vi "Prime95BCameraSimpleOperation.vi"(8 "error in (no error)":errorcluster, 11 "Config In":T3 {"Hardware Configuration"."Lasers Configuration"."SettingValues"."785 Power" format="%.1f"; "Hardware Configuration"."Lasers Configuration"."SettingValues"."647 Power" format="%.1f"; "Hardware Configuration"."Lasers Configuration"."SettingValues"."561 Power" format="%.1f"}) -> (0 "error out":errorcluster, 3 "Config Out":T3 {"Hardware Configuration"."Lasers Configuration"."SettingValues"."785 Power" format="%.1f"; "Hardware Configuration"."Lasers Configuration"."SettingValues"."647 Power" format="%.1f"; "Hardware Configuration"."Lasers Configuration"."SettingValues"."561 Power" format="%.1f"})   [LabVIEW 2019]
uses:
  Settings/System Running Settings.ctl
  HardwareAdapter/Support/Hardware Configuration.ctl
  HardwareAdapter/Support/Camera Configuration.ctl
  E:/DevHardSoftware/MMicroscopy/HardwareAdapter/Camera/Dependencies/PVCamNET.dll
  HardwareAdapter/Camera/Dependencies/PVCamNET.dll
  <vilib>/vision/Image Controls.llb/IMAQ Image.ctl
  E:/DevHardSoftware/MMicroscopy/HardwareAdapter/Lasers/Dependencies/Oxxius_Boxx.dll
  HardwareAdapter/Lasers/Dependencies/Oxxius_Boxx.dll
  Logging/Logging Configuration.ctl
  controls/DeviceStatusCtl.ctl
  controls/CallBack Refs.ctl
  Logging/Logging.lvlib
  Settings/Settings.lvlib
panel:
  in  "Image Type":T1 items=["Grayscale (U8)", "Grayscale (I16)", "Grayscale (SGL)", "Complex (CSG)", "RGB (U32)", "HSL (U32)", "RGB (U64)", "Grayscale (U16)"]
  out "Image 2":T2(plugin-control)
  in  "start":bool
  out "BitDepth":u32
  in  "stop 2":bool
  in  "Exposure time":dbl=30.0
  in  "stop":bool
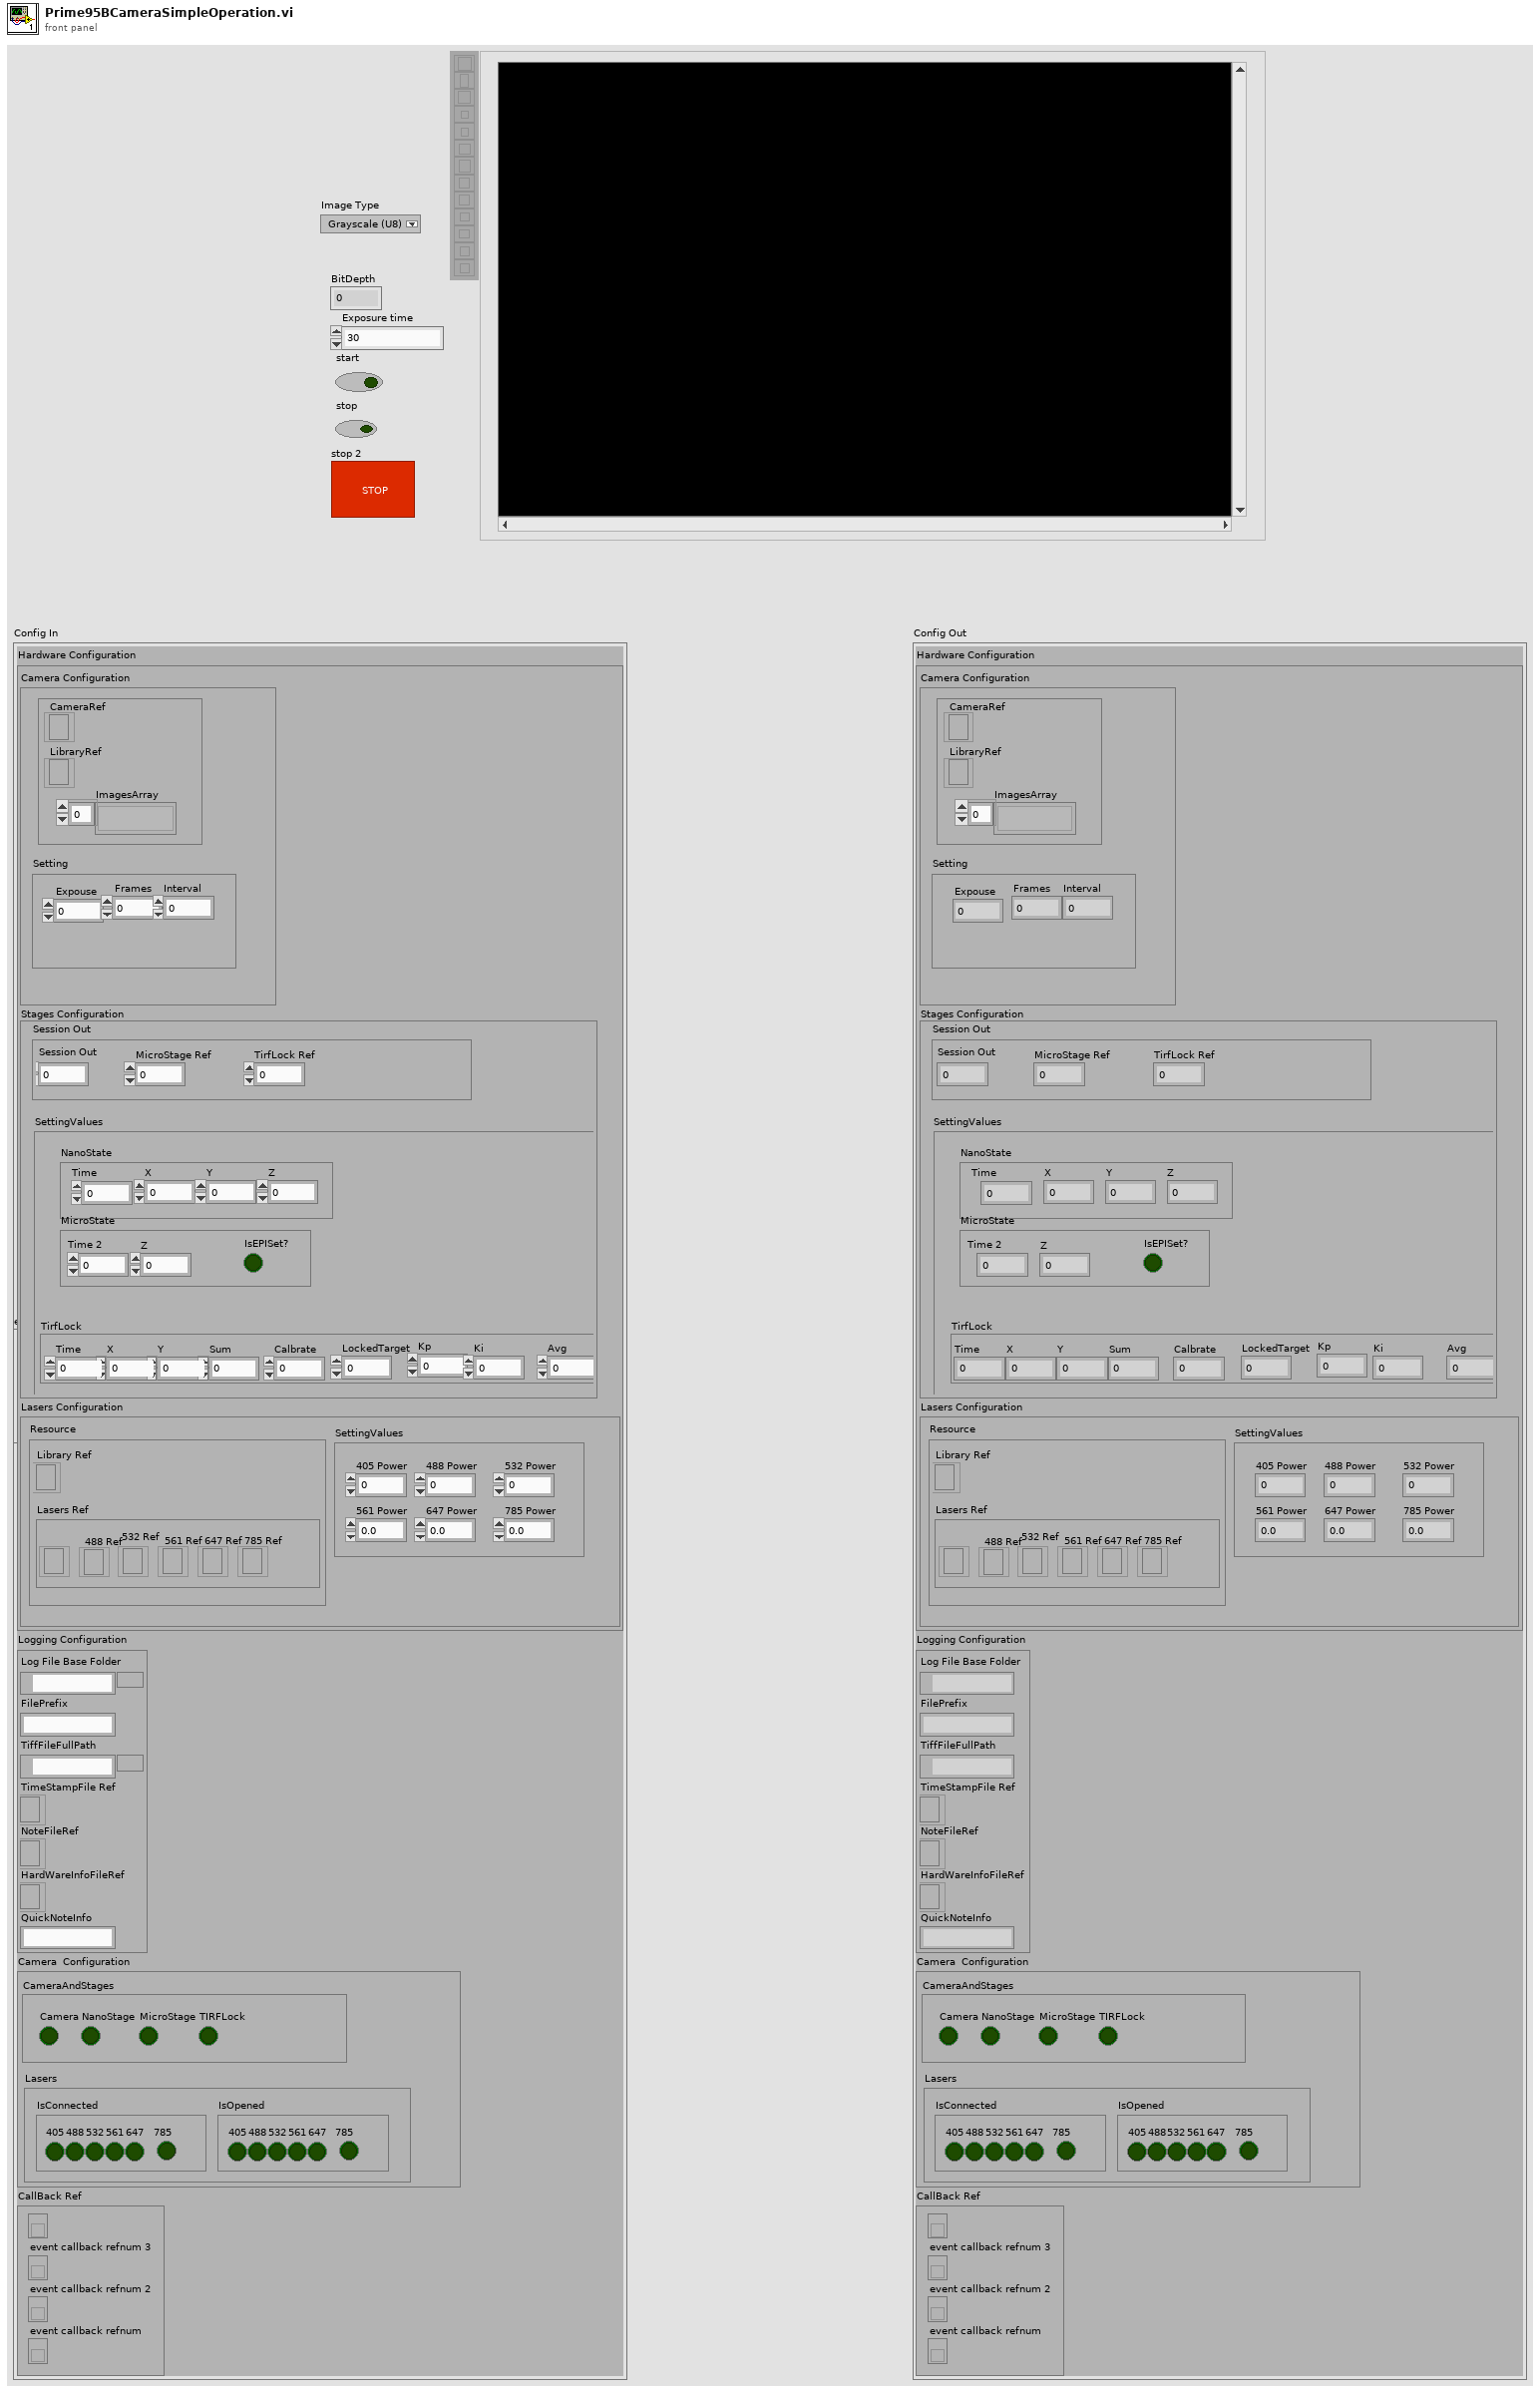
[diagram p1: front panel]
types:
  T1 = typedef "Image Type" = u32
  T2 = typedef "IMAQ Image.ctl" = refnum<image>
  T3 = typedef "Settings.lvlib/System Running Settings.ctl" = cluster{"Hardware Configuration":T4, "Logging Configuration":T6, "HardWare Status":cluster{"CameraAndStages":T7, "Lasers":cluster{"IsConnected":cluster{"405":bool, "488":bool, "532":bool, "561":bool, "647":bool, "785":bool}, "IsOpened":cluster{"405":bool, "488":bool, "532":bool, "561":bool, "647":bool, "785":bool}}}, "CallBack Ref":T8}
  T4 = typedef "Hardware Configuration.ctl" = cluster{"Camera Configuration":T5, "Stages Configuration":cluster{"Resource":cluster{"NanoStage Ref":i32, "MicroStage Ref":i32, "TirfLock Ref":i32}, "SettingValues":cluster{"NanoState":cluster{"Time":dbl, "X":dbl, "Y":dbl, "Z":dbl}, "MicroState":cluster{"Time 2":dbl, "Z":dbl, "IsEPISet?":bool}, "TirfLock":cluster{"Time":dbl, "X":dbl, "Y":dbl, "Sum":dbl, "Calbrate":dbl, "LockedTarget":dbl, "Kp":dbl, "Ki":dbl, "Avg":dbl}}}, "Lasers Configuration":cluster{"SettingValues":cluster{"405 Power":sgl, "488 Power":sgl, "532 Power":sgl, "561 Power":sgl, "647 Power":sgl, "785 Power":sgl}, "Resource":cluster{"Library Ref":refnum<k24>, "Lasers Ref":cluster{"405 Ref":refnum<k24>, "488 Ref":refnum<k24>, "532 Ref":refnum<k24>, "561 Ref":refnum<k24>, "647 Ref":refnum<k24>, "785 Ref":refnum<k24>}}}}
  T5 = typedef "Camera Configuration.ctl" = cluster{"Setting":cluster{"Expouse":dbl, "Frames":dbl, "Interval":dbl}, "Resource":cluster{"CameraRef":refnum<k24>, "LibraryRef":refnum<k24>, "ImagesArray":T2[]}}
  T6 = typedef "Logging.lvlib/Logging Configuration.ctl" = cluster{"Log File Base Folder":path, "FilePrefix":string, "TiffFileFullPath":path, "TimeStampFile Ref":refnum<file>, "NoteFileRef":refnum<file>, "HardWareInfoFileRef":refnum<file>, "QuickNoteInfo":string}
  T7 = typedef "DeviceStatusCtl.ctl" = cluster{"Camera":bool, "NanoStage":bool, "MicroStage":bool, "TIRFLock":bool}
  T8 = typedef "CallBack Refs.ctl" = cluster{"event callback refnum":refnum<k27>, "event callback refnum 2":refnum<k27>, "event callback refnum 3":refnum<k27>, "event callback refnum 4":refnum<k27>}
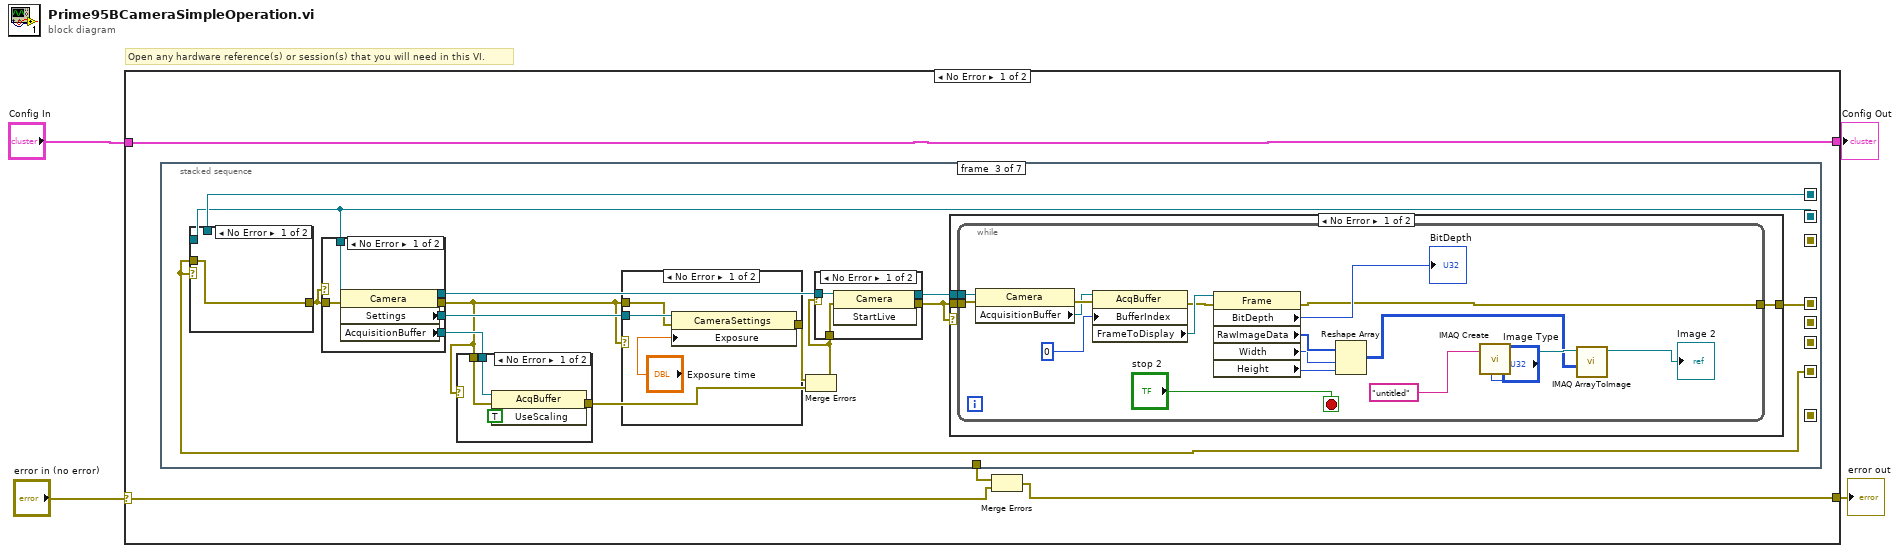
[diagram p0: block diagram]
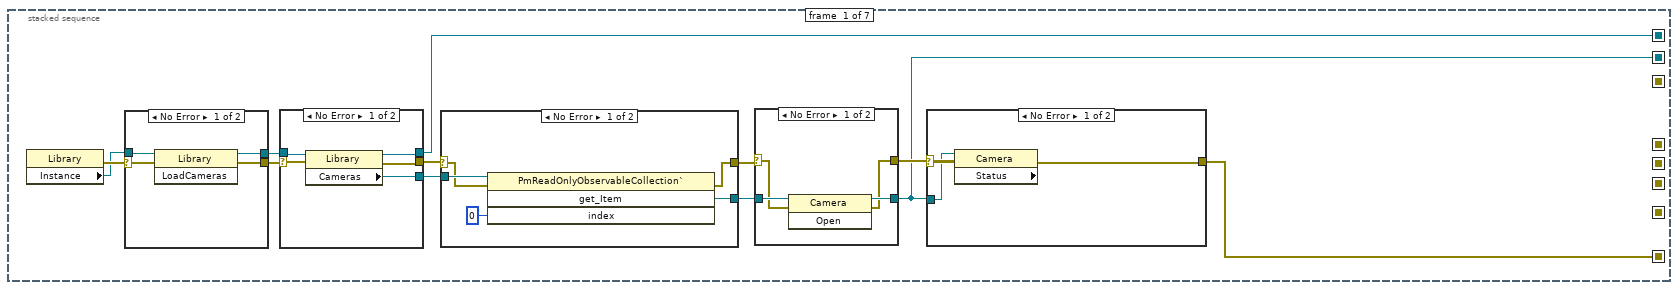
[diagram p2: hidden frame]
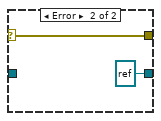
[diagram p4: hidden frame]
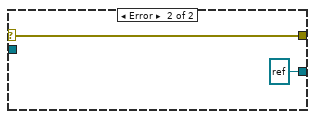
[diagram p5: hidden frame]
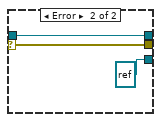
[diagram p6: hidden frame]
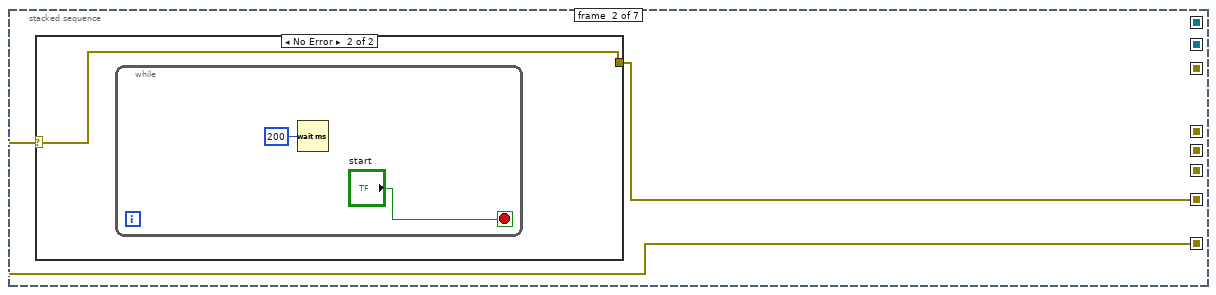
[diagram p8: hidden frame]
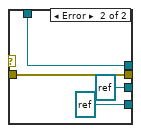
[diagram p13: hidden frame]
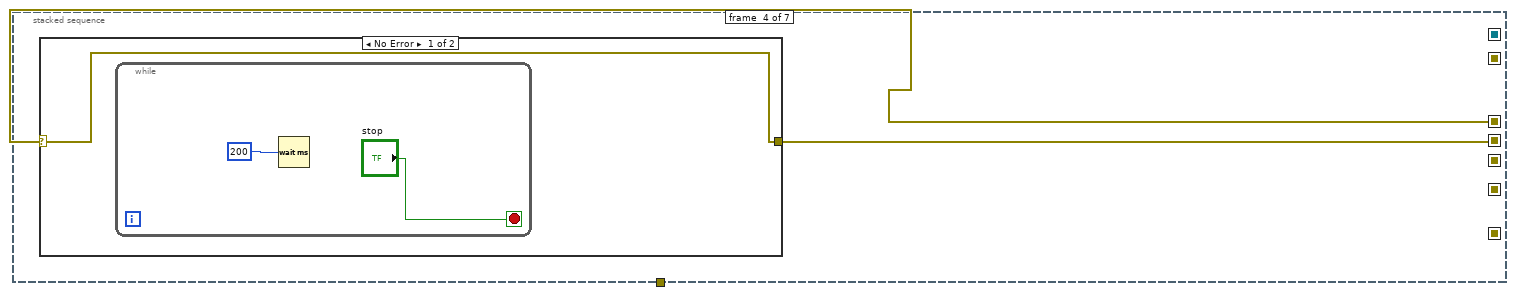
[diagram p16: hidden frame]
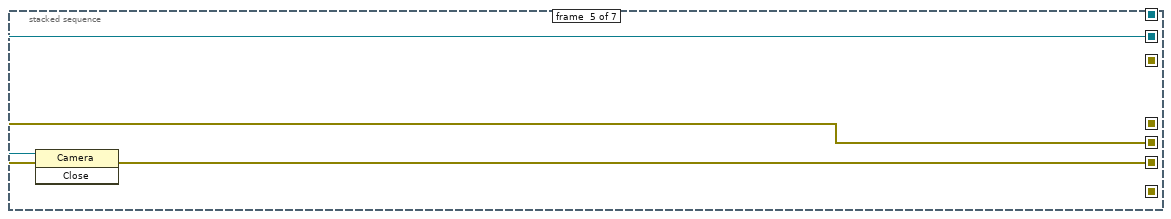
[diagram p18: hidden frame]
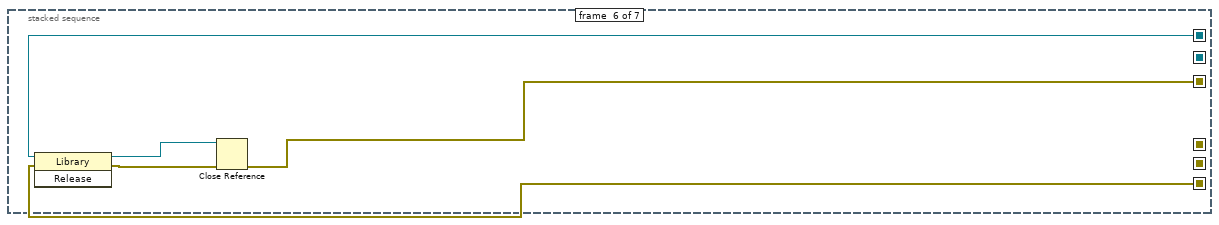
[diagram p19: hidden frame]
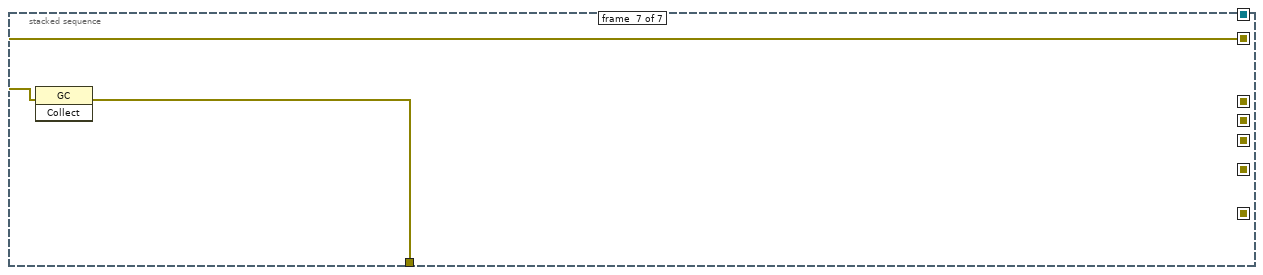
[diagram p20: hidden frame]
diagram:
  # "Open any hardware reference(s) or session(s) that you will need in this VI."
  n1 = case shown="No Error" "error in (no error)" {
    selector: "error in (no error)" -> [w6 w138]
    tunnel: [w5 w138] -> w3
    tunnel: "Config In" -> [w8 w139]
    tunnel: [w8 w139] -> w1
    frame No Error {
      n2 = stacked-sequence {
        seq-local: [w9 _ _ _ _ _ _] -> [_ w53 _ _ _ _ _]
        seq-local: [w10 _ _ _ _ _ _] -> [_ _ w68 _ w130 _ _]
        seq-local: [w12 _ _ _ _ _ _] -> [_ _ w71 _ _ w134 _]
        seq-local: [_ _ w65 _ _ _ _] -> [_ _ _ w123 _ _ _]
        seq-local: [_ _ _ _ w129 _ _] -> [_ _ _ _ _ w133 _]
        seq-local: [_ _ _ _ _ w131 _] -> [_ _ _ _ _ _ w137]
        seq-local: [_ w52 _ _ _ _ _] -> [_ _ w62 _ _ _ _]
        seq-local: [_ _ _ w122 _ _ _] -> [_ _ _ _ w128 _ _]
        tunnel: [_ _ _ _ _ _ w136] -> w7
        frame #0 {
          n3 = property class="Library"() -> (error out=w20:errorcluster, "Instance"=w17:refnum<k24>)  [unwired: 2 in, 1 out]
          n4 = case shown="No Error" w20 {
            selector: w20 -> [w47 w51]
            tunnel: [w48 w51] -> w18
            tunnel: [w49 w50] -> w19
            tunnel: w17 -> [w46 w50]
            frame No Error {
              n5 = invoke class="Library" method="LoadCameras"(reference=w46, error in=w47) -> (reference out=w49:refnum<k24>, error out=w48:errorcluster)  [unwired: 1 in, 1 out]
            }
            frame Error {
            }
          }
          n6 = case shown="No Error" w18 {
            selector: w18 -> [w42 w45]
            tunnel: [w39 w45] -> w14
            tunnel: w19 -> [w41 w44]
            tunnel: [w40 w44] -> w12
            tunnel: [w38 refnum<k24> refnum ("Cameras")] -> w16
            frame No Error {
              n7 = property class="Library"(reference=w41, error in=w42) -> (reference out=w40:refnum<k24>, error out=w39:errorcluster, "Cameras"=w38:refnum<k24>)
            }
            frame Error {
            }
          }
          n8 = case shown="No Error" w14 {
            selector: w14 -> [w32 w37]
            tunnel: w16 -> [w35 _]
            tunnel: [w33 refnum<k24> refnum ("get_Item")] -> w15
            tunnel: [w31 w37] -> w13
            frame No Error {
              n9 = invoke class="PmReadOnlyObservableCollection`" method="get_Item"(reference=w35, error in=w32, "index"=0) -> (error out=w31:errorcluster, "get_Item"=w33:refnum<k24>)  [unwired: 1 in, 2 out]
            }
            frame Error {
            }
          }
          n10 = case shown="No Error" w13 {
            selector: w13 -> [w26 w30]
            tunnel: [w25 w30] -> w11
            tunnel: w15 -> [w28 _]
            tunnel: [w27 refnum<k24> refnum ("get_Item")] -> w10
            frame No Error {
              n11 = invoke class="Camera" method="Open"(reference=w28, error in=w26) -> (reference out=w27:refnum<k24>, error out=w25:errorcluster)  [unwired: 1 in, 1 out]
            }
            frame Error {
            }
          }
          n12 = case shown="No Error" w11 {
            selector: w11 -> [w22 w24]
            tunnel: [w21 w24] -> w9
            tunnel: w10 -> [w23 _]
            frame No Error {
              n13 = property class="Camera" props=["Status"](reference=w23, error in=w22) -> (error out=w21:errorcluster)  [unwired: 2 out]
            }
            frame Error {
            }
          }
        }
        frame #1 {
          n14 = case shown="No Error" w53 {
            selector: w53 -> [w54 w55]
            tunnel: [w54 w55] -> w52
            frame Error {
            }
            frame No Error {
              n15 = while {
                stop <- "start" stop-if-true
                n16 = Wait (ms)(milliseconds to wait=u32 200) -> ()  [unwired: 1 out]
              }
            }
          }
        }
        frame #2 {
          n17 = case shown="No Error" w62 {
            tunnel: w71 -> [_ _]
            tunnel: [w98 w99] -> w61
            tunnel: w68 -> [_ _]
            tunnel: w62 -> [w98 w99]
            frame No Error {
            }
            frame Error {
            }
          }
          n18 = case shown="No Error" w61 {
            tunnel: [w93 refnum<k24> refnum ("Settings")] -> w70
            tunnel: [w92 refnum<k24> refnum ("AcquisitionBuffer")] -> w69
            tunnel: w61 -> [w91 w97]
            tunnel: w68 -> [w90 w96]
            tunnel: [w89 w96] -> w67
            tunnel: [w88 w97] -> w60
            frame No Error {
              n19 = property class="Camera"(reference=w90, error in=w91) -> (reference out=w89:refnum<k24>, error out=w88:errorcluster, "Settings"=w93:refnum<k24>, "AcquisitionBuffer"=w92:refnum<k24>)
            }
            frame Error {
            }
          }
          n20 = case shown="No Error" w60 {
            selector: w60 -> [_ w87]
            tunnel: w69 -> [w86 _]
            tunnel: w60 -> [w84 _]
            tunnel: [w83 w87] -> w63
            frame No Error {
              n21 = property class="AcqBuffer"(reference=w86, error in=w84, "UseScaling"=TRUE) -> (error out=w83:errorcluster)  [unwired: 1 out]
            }
            frame Error {
            }
          }
          n22 = case shown="No Error" w60 {
            tunnel: w70 -> [w80 _]
            tunnel: [w79 w82] -> w64
            tunnel: w60 -> [w78 w82]
            frame No Error {
              n23 = property class="CameraSettings"(reference=w80, error in=w78, "Exposure"="Exposure time") -> (error out=w79:errorcluster)  [unwired: 1 out]
            }
            frame Error {
            }
          }
          n24 = Merge Errors(w64, w63) -> (w59:errorcluster)
          n25 = case shown="No Error" w59 {
            selector: w59 -> [_ w77]
            tunnel: w67 -> [w75 w76]
            tunnel: [w74 w77] -> w58
            tunnel: [w73 w76] -> w66
            tunnel: w59 -> [w72 _]
            frame No Error {
              n26 = invoke class="Camera" method="StartLive"(reference=w75, error in=w72) -> (reference out=w73:refnum<k24>, error out=w74:errorcluster)  [unwired: 1 in, 1 out]
            }
            frame Error {
            }
          }
          n27 = case shown="No Error" w58 {
            tunnel: w58 -> [w102 w121]
            tunnel: w66 -> [w101 _]
            tunnel: [w100 w121] -> w65
            frame No Error {
              n28 = while {
                tunnel: w102 -> [w111]
                tunnel: w101 -> [w120]
                tunnel: [w112] -> w100
                stop <- "stop 2" stop-if-true
                n29 = property class="Camera"(reference=w120, error in=w111) -> (error out=w119:errorcluster, "AcquisitionBuffer"=w118:refnum<k24>)  [unwired: 1 out]
                n30 = property class="AcqBuffer"(reference=w118, error in=w119, "BufferIndex"=0) -> (error out=w115:errorcluster, "FrameToDisplay"=w116:refnum<k24>)  [unwired: 1 out]
                n31 = property class="Frame"(reference=w116, error in=w115) -> (error out=w112:errorcluster, "BitDepth"=→"BitDepth":u32, "RawImageData"=w110:i16[], "Width"=w109:u32, "Height"=w108:u32)  [unwired: 1 out]
                n32 = Reshape Array "Reshape Array"(w110, w109, w108) -> (w104:i16[][])
                n33 = call "IMAQ Create"("Image Name"="untitled", "Image Type"="Image Type") -> ("New Image"=w105:T2)  [unwired: 2 in, 2 out]
                n34 = call "IMAQ ArrayToImage"("Image Pixels (I16)"=w104, "Image"=w105) -> ("Image Out"=→"Image 2":T2)  [unwired: 8 in, 1 out]
              }
            }
            frame Error {
            }
          }
        }
        frame #3 {
          n35 = case shown="No Error" w123 {
            selector: w123 -> [w124 w127]
            tunnel: [w124 w127] -> w122
            frame No Error {
              n36 = while {
                stop <- "stop" stop-if-true
                n37 = Wait (ms)(milliseconds to wait=u32 200) -> ()  [unwired: 1 out]
              }
            }
            frame Error {
            }
          }
        }
        frame #4 {
          n38 = invoke class="Camera" method="Close"(reference=w130, error in=w128) -> (error out=w129:errorcluster)  [unwired: 1 in, 2 out]
        }
        frame #5 {
          n39 = invoke class="Library" method="Release"(reference=w134, error in=w133) -> (reference out=w135:refnum<k24>, error out=w132:errorcluster)  [unwired: 1 in, 1 out]
          n40 = Close Reference(reference=w135, error in (no error)=w132) -> (error out=w131:errorcluster)
        }
        frame #6 {
          n41 = invoke class="GC" method="Collect"(error in=w137) -> (error out=w136:errorcluster)  [unwired: 2 in, 2 out]
        }
      }
      n42 = Merge Errors(w7, w6) -> (w5:errorcluster)
    }
    frame Error {
    }
  }
  "error out" <- w3
  "Config Out" <- w1
